vi "Write directory.vi"(8 "error in (no error)":errorcluster, 11 "Log File in":refnum<class "Events Log File.lvclass">) -> (0 "error out":errorcluster, 3 "Log File out":refnum<class "Events Log File.lvclass">)   [LabVIEW 2018, in "Events Log File.lvclass"]
uses:
  Events Log File.lvclass
  Events Log File.lvclass/Events Log File.ctl
  <vilib>/Utility/config.llb/Read Key (String).vi
  <vilib>/Utility/config.llb/Read Key (U32).vi
  <vilib>/Utility/config.llb/NI_LVConfig.lvlib
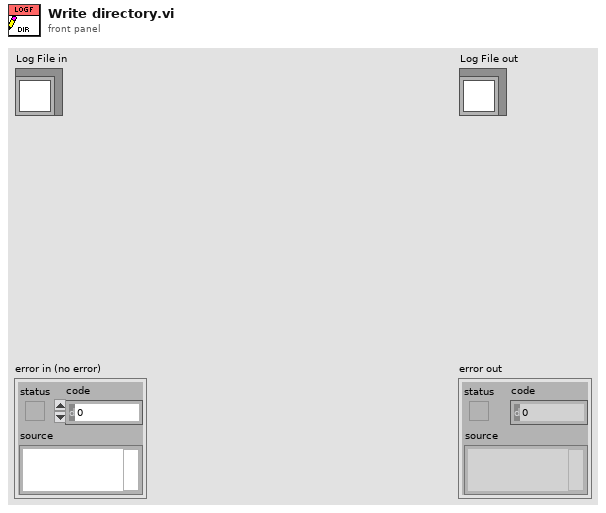
[diagram p1: front panel]
types:
  T1 = typedef "NI_LVConfig.lvlib/Config Data RefNum.ctl" = refnum<k1>
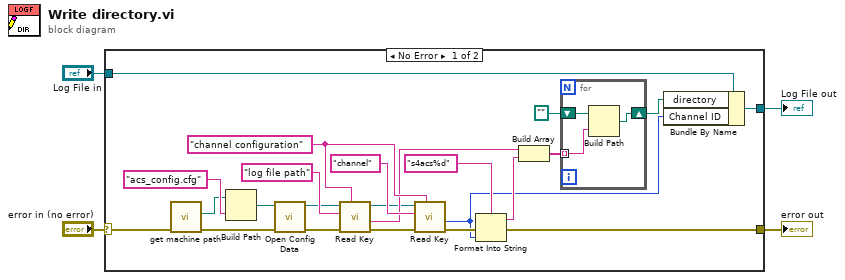
[diagram p0: block diagram]
diagram:
  n1 = case shown="No Error" "error in (no error)" {
    selector: "error in (no error)" -> [w10 w31]
    tunnel: [w7 w31] -> w3
    tunnel: [w8 w32] -> w1
    tunnel: "Log File in" -> [w9 w32]
    frame No Error {
      w21 = "channel configuration"
      n2 = call "get machine path.vi"("error in (no error) 2"=w10) -> ("error in (no error)"=w25:errorcluster, "machine path"=w24:path)  [unwired: 9 in]
      n3 = Build Path(base path=w24, name or relative path="acs_config.cfg") -> (appended path=w27:path)
      n4 = call <vilib>:"Open Config Data.vi"("error in (no error)"=w25, "configuration file path"=w27) -> ("error out"=w20:errorcluster, "refnum"=w12:T1)  [unwired: 7 in, 1 out]
      n5 = call-poly <vilib>:"Read Key.vi"("section"=w21, "error in (no error)"=w20, "key"="log file path", "refnum"=w12) -> ("error out"=w19:errorcluster, "value"=w18:string, "refnum out"=w11:T1)  [unwired: 4 in, 1 out]
      n6 = call-poly <vilib>:"Read Key.vi"("section"=w21, "error in (no error)"=w19, "key"="channel", "refnum"=w11) -> ("error out"=w15:errorcluster, "value"=w5:u32)  [unwired: 4 in, 2 out]
      n7 = Format Into String(format string="s4acs%d", error in=w15, w5) -> (resulting string=w16:string, error out=w7:errorcluster)  [unwired: 1 in]
      n8 = Build Array(w18, w16) -> (w13:string[])
      n9 = for {
        shift-right: [w30] -> w6
        shift-left: path "" -> [w29]
        tunnel: w13 -> [w28] mode=indexing
        n10 = Build Path(base path=w29, name or relative path=w28) -> (appended path=w30:path)
      }
      n11 = Bundle By Name(cluster=w9, "directory"=w6, "Channel ID"=w5) -> (w8:refnum<class "Events Log File.lvclass">)
    }
    frame Error {
    }
  }
  "error out" <- w3
  "Log File out" <- w1
